vi "save_expSD.vi"(1 "exp selected":i32, 3 "error in (no error)":errorcluster, 4 "Group":u16, 5 "save Radio Buttons":enum32{"Automatic", "User-def"}(ring), 6 "Experiments groups in":refnum<class "Experiments_group.lvclass">[](array[class])) -> (0 "error out":errorcluster, 2 "Experiments groups out":refnum<class "Experiments_group.lvclass">[](array[class]))   [LabVIEW 2015]
uses:
  Classes/Experiments_group.lvclass
  Classes/Experiment.lvclass
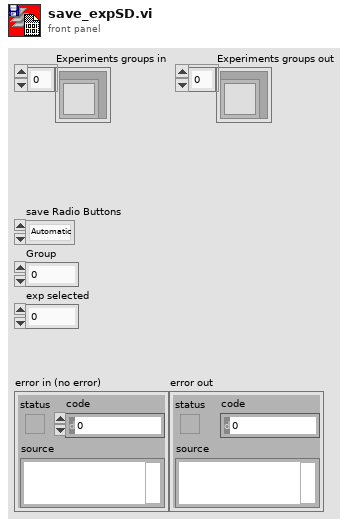
[diagram p1: front panel]
types:
  T1 = enum16{"open", "replace", "create", "open or create", "replace or create", "replace or create with confirmation"}
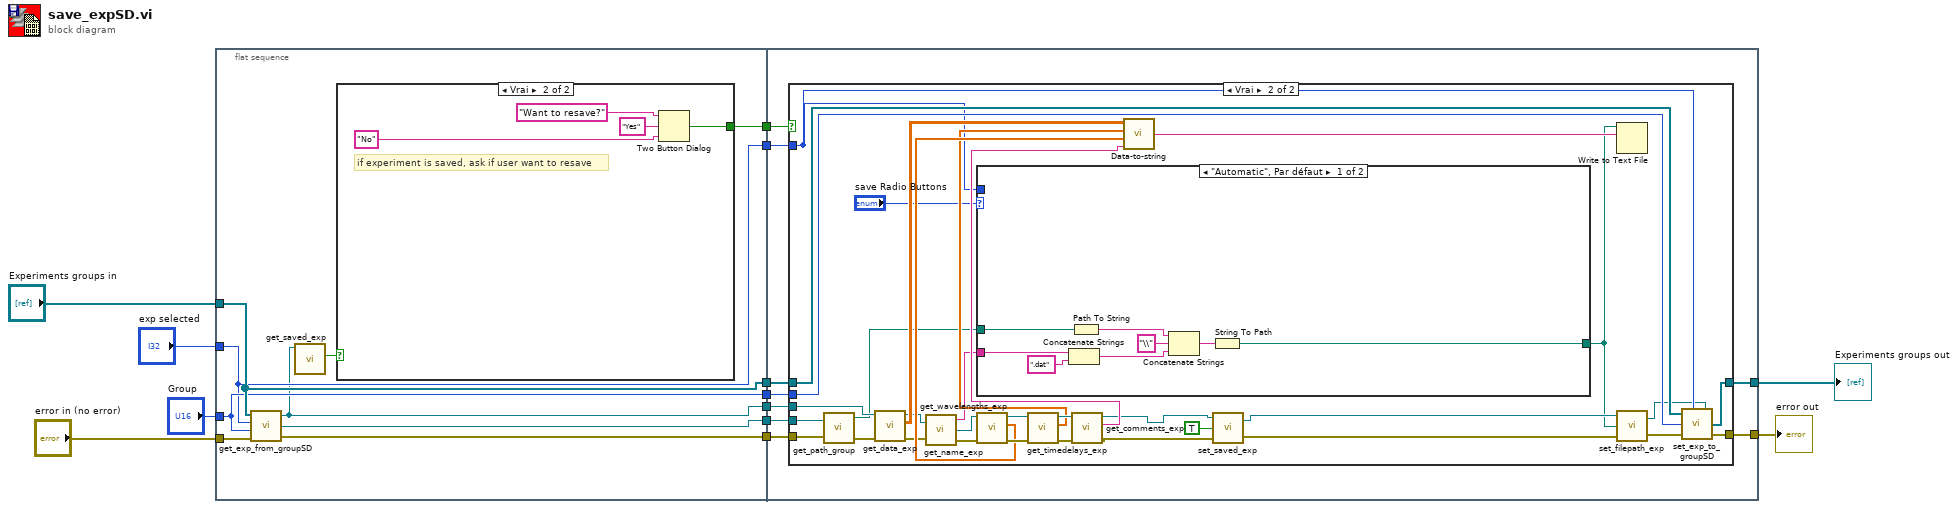
[diagram p0: block diagram]
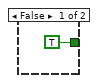
[diagram p2: hidden frame]
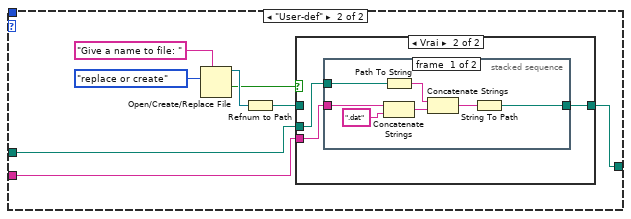
[diagram p4: hidden frame]
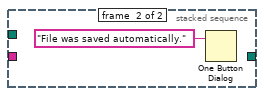
[diagram p6: hidden frame]
diagram:
  n1 = flat-sequence {
    tunnel: "Experiments groups in" -> [w21]
    tunnel: "error in (no error)" -> [w17]
    tunnel: [w22] -> w13
    tunnel: [w20] -> w12
    tunnel: [w19] -> w11
    tunnel: [w21] -> w10
    tunnel: [w16] -> w9
    tunnel: "Group" -> [w20]
    tunnel: "exp selected" -> [w18]
    tunnel: [w18] -> w2
    tunnel: [w14] -> w1
    tunnel: w13 -> [w36]
    tunnel: w12 -> [w30]
    tunnel: w11 -> [w35]
    tunnel: w10 -> [w34]
    tunnel: [w33] -> w5
    tunnel: [w32] -> w6
    tunnel: w9 -> [w31]
    tunnel: w2 -> [w29]
    tunnel: w1 -> [w28]
    frame #0 {
      n2 = call "get_exp_from_groupSD.vi"("error in (no error)"=w17, "group"=w20, "exp selected"=w18, "Experiments groups"=w21) -> ("error out"=w19:errorcluster, "Group"=w14:refnum<class "Experiments_group.lvclass">, "Experiment out"=w16:refnum<class "Experiment.lvclass">)
      n3 = call-dynamic "get_saved_exp.vi"("Experiment.lvclass in"=w16) -> ("Saved"=w15:bool)  [unwired: 8 in, 2 out]
      n4 = case shown="Vrai" w15 {
        tunnel: [TRUE ("T button?") w24] -> w22
        frame False {
        }
        frame True {
          # "if experiment is saved, ask if user want to resave"
          n5 = Two Button Dialog(message="Want to resave?", 1:"No" ("F button name (\"Cancel\")"), 2:"Yes" ("T button name (\"OK\")")) -> (T button?=w24:bool)
        }
      }
    }
    frame #1 {
      n6 = case shown="Vrai" w36 {
        tunnel: w35 -> [w38 w65]
        tunnel: [w38 w54] -> w32
        tunnel: w34 -> [w37 w56]
        tunnel: [w37 w55] -> w33
        tunnel: w31 -> [_ w64]
        tunnel: w30 -> [_ w57]
        tunnel: w29 -> [_ w53]
        tunnel: w28 -> [_ w52]
        frame False {
        }
        frame True {
          n7 = call-dynamic "get_path_group.vi"("Experiments_group.lvclass in"=w52, "error in (no error)"=w65) -> ("Path"=w58:path, "error out"=w67:errorcluster)  [unwired: 1 out]
          n8 = call-dynamic "get_data_exp.vi"("error in (no error)"=w67, "Experiment.lvclass in"=w64) -> ("error out"=w51:errorcluster, "Data"=w63:dbl[][], "Experiment.lvclass out"=w48:refnum<class "Experiment.lvclass">)  [unwired: 7 in]
          n9 = call-dynamic "get_name_exp.vi"("Experiment.lvclass in"=w48, "error in (no error)"=w51) -> ("Exp name"=w47:string, "Experiment.lvclass out"=w49:refnum<class "Experiment.lvclass">, "error out"=w50:errorcluster)
          n10 = case shown="\"Automatic\", Par défaut" "save Radio Buttons" {
            tunnel: w58 -> [w78 w81]
            tunnel: w53 -> [_ _]
            tunnel: [w75 w83] -> w41
            tunnel: w47 -> [w72 w80]
            frame "Automatic", Default {
              n11 = Concatenate Strings(w72, ".dat" ("string")) -> (w74:string)
              n12 = Path To String(path=w78) -> (string=w77:string)
              n13 = Concatenate Strings(w77, "\\" ("string"), w74) -> (w76:string)
              n14 = String To Path(string=w76) -> (path=w75:path)
            }
            frame "User-def" {
              n15 = Open/Create/Replace File(prompt="Give a name to file: ", operation (0:open)=T1."replace or create") -> (refnum out=w85:refnum<file>, cancelled=w84:bool)  [unwired: 4 in, 1 out]
              n16 = Refnum to Path(1:w85) -> (0:w82:path)
              n17 = case shown="Vrai" w84 {
                tunnel: [w88 w91] -> w83
                tunnel: w82 -> [w88 _]
                tunnel: w81 -> [_ w90]
                tunnel: w80 -> [_ w89]
                frame False {
                }
                frame True {
                  n18 = stacked-sequence {
                    tunnel: [w94 _] -> w91
                    tunnel: w90 -> [w93 _]
                    tunnel: w89 -> [w92 _]
                    frame #0 {
                      n19 = Path To String(path=w93) -> (string=w97:string)
                      n20 = Concatenate Strings(w92, ".dat" ("string")) -> (w96:string)
                      n21 = Concatenate Strings(w97, w96) -> (w95:string)
                      n22 = String To Path(string=w95) -> (path=w94:path)
                    }
                    frame #1 {
                      n23 = One Button Dialog(message="File was saved automatically.") -> ()  [unwired: 1 in, 1 out]
                    }
                  }
                }
              }
            }
          }
          n24 = call-dynamic "get_wavelengths_exp.vi"("error in (no error)"=w50, "Experiment.lvclass in"=w49) -> ("error out"=w69:errorcluster, "wavelengths"=w62:dbl[], "Experiment.lvclass out"=w68:refnum<class "Experiment.lvclass">)  [unwired: 7 in]
          n25 = call-dynamic "get_timedelays_exp.vi"("error in (no error)"=w69, "Experiment.lvclass in"=w68) -> ("error out"=w70:errorcluster, "timedelays"=w61:dbl[], "Experiment.lvclass out"=w71:refnum<class "Experiment.lvclass">)  [unwired: 7 in]
          n26 = call-dynamic "get_comments_exp.vi"("error in (no error)"=w70, "Experiment.lvclass in"=w71) -> ("error out"=w39:errorcluster, "Comments"=w60:string, "Experiment.lvclass out"=w40:refnum<class "Experiment.lvclass">)  [unwired: 7 in]
          n27 = call "Data-to-string.vi"("string"=w60, "wavelength"=w62, "timedelay"=w61, "DATA"=w63) -> ("resulted string"=w59:string)
          n28 = call-dynamic "set_saved_exp.vi"("error in (no error)"=w39, "Saved"=TRUE, "Experiment.lvclass in"=w40) -> ("error out"=w43:errorcluster, "Experiment.lvclass out"=w45:refnum<class "Experiment.lvclass">)
          n29 = Write to Text File(file (use dialog)=w41, text=w59) -> ()  [unwired: 2 in, 3 out]
          n30 = call-dynamic "set_filepath_exp.vi"("error in (no error)"=w43, "FilePath"=w41, "Experiment.lvclass in"=w45) -> ("error out"=w42:errorcluster, "Experiment.lvclass out"=w44:refnum<class "Experiment.lvclass">)
          n31 = call "set_exp_to_groupSD.vi"("Experiments groups"=w56, "exp selected"=w53, "group"=w57, "error in (no error)"=w42, "Experiment in"=w44) -> ("Experiments groups out"=w55:refnum<class "Experiments_group.lvclass">[], "error out"=w54:errorcluster)  [unwired: 1 in]
        }
      }
    }
  }
  "error out" <- w6
  "Experiments groups out" <- w5
